vi "notifier.vi"() -> ()   [LabVIEW 2018]
panel:
  out "input data":dbl(graph)
  in  "정지":bool
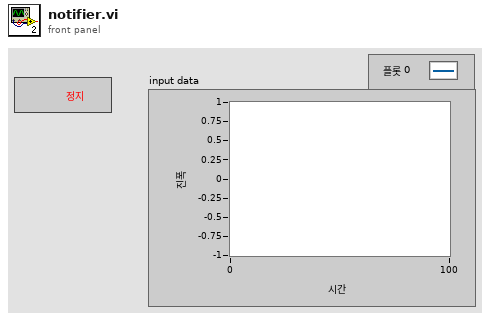
[diagram p1: front panel]
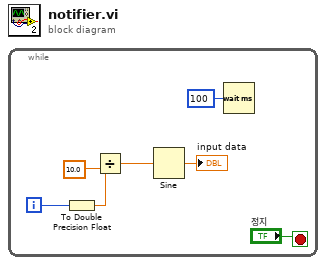
[diagram p0: block diagram]
diagram:
  n1 = while {
    i -> [w7]
    stop <- "정지" stop-if-true
    n2 = To Double Precision Float(number=w7) -> (double precision float=w6:dbl)
    n3 = Divide(x=w6, y=10.0) -> (x/y=w4:dbl)
    n4 = Sine(x=w4) -> (sin(x)=→"input data":dbl)
    n5 = Wait (ms)(milliseconds to wait=u32 100 ("대기 시간 (ms)")) -> ()  [unwired: 1 out]
  }
